vi "SAVE_TCP_CONFIG.vi"(10 "PortNumber":u16=25534, 11 "IP Addr":string="172.22.11.2") -> (0 "에러 출력":errorcluster)   [LabVIEW 2023]
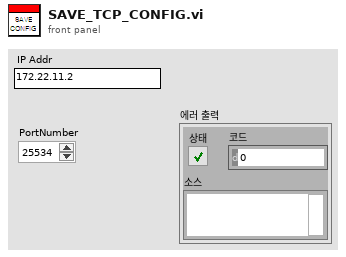
[diagram p1: front panel]
types:
  T1 = enum16{"open", "replace", "create", "open or create", "replace or create", "replace or create with confirmation"}
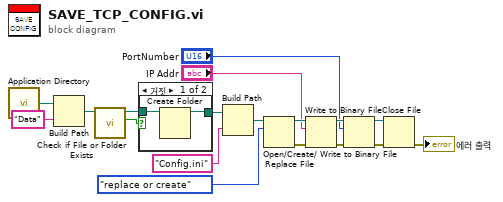
[diagram p0: block diagram]
diagram:
  n1 = call <vilib>:"Application Directory.vi"() -> ("Application Directory"=w15:path)
  n2 = Build Path(base path=w15, name or relative path="Data" ("이름 또는 상대 경로")) -> (appended path=w17:path)
  n3 = call <vilib>:"Check if File or Folder Exists.vi"("path"=w17) -> ("file or folder exists?"=w1:bool, "dup path"=w18:path)  [unwired: 8 in, 1 out]
  n4 = case shown="거짓" w1 {
    tunnel: w18 -> [w20 w21]
    tunnel: [w19 w21] -> w14
    frame False {
      n5 = Create Folder(path (use dialog)=w20) -> (created path=w19:path)  [unwired: 2 in, 2 out]
    }
    frame True {
    }
  }
  n6 = Build Path(base path=w14, name or relative path="Config.ini" ("이름 또는 상대 경로")) -> (appended path=w13:path)
  n7 = Open/Create/Replace File(file path (use dialog)=w13, operation (0:open)=T1."replace or create" ("동작(0:open)")) -> (refnum out=w11:refnum<file>, error out=w10:errorcluster)  [unwired: 4 in, 1 out]
  n8 = Write to Binary File(file (use dialog)=w11, data="IP Addr", error in=w10) -> (refnum out=w8:refnum<file>, error out=w7:errorcluster)  [unwired: 3 in, 1 out]
  n9 = Write to Binary File(file (use dialog)=w8, data="PortNumber", error in=w7) -> (refnum out=w3:refnum<file>, error out=w2:errorcluster)  [unwired: 3 in, 1 out]
  n10 = Close File(refnum=w3, error in=w2) -> (error out=→"에러 출력":errorcluster)  [unwired: 1 out]
